vi "Multi-FuncGlobal.vi"(11 "Operation and Data In":T1) -> (1 "Time Out":dbl, 2 "Numeric Out":dbl, 3 "String Out":string)   [LabVIEW 2012]
doc: "This is a Multi-Functional Global Variable, meaning it can save a number, string, and also get the elapsed time since its time was last checked."
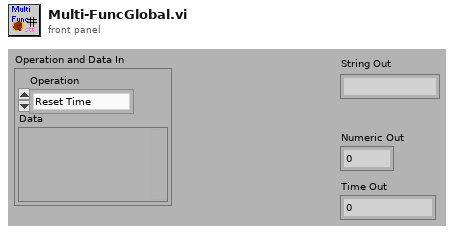
[diagram p1: front panel]
types:
  T1 = cluster{"Operation":enum16{"Reset Time", "Set String", "Set Number", "Get Elapsed Time", "Get String", "Get Number"}, "Data":variant}
  T2 = enum16{"Reset Time", "Set String", "Set Number", "Get Elapsed Time", "Get String", "Get Number"}
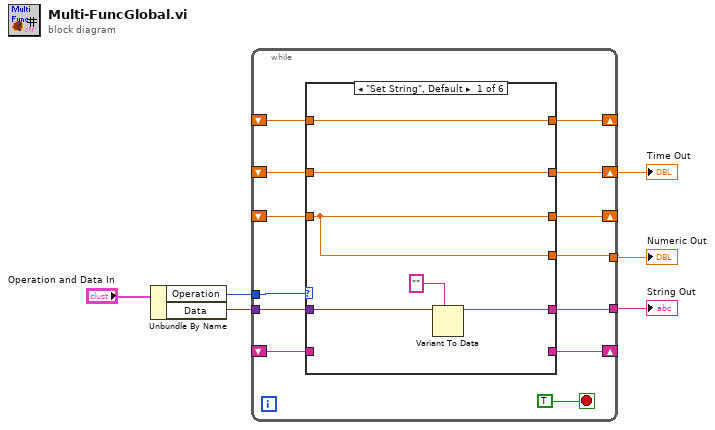
[diagram p0: block diagram]
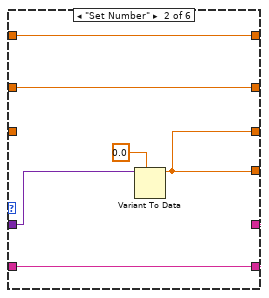
[diagram p2: hidden frame]
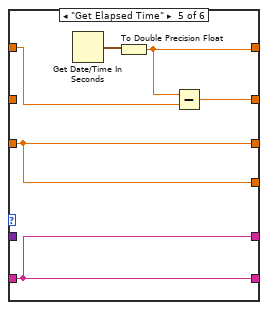
[diagram p5: hidden frame]
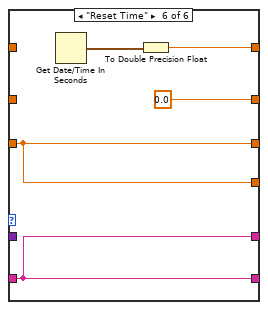
[diagram p6: hidden frame]
diagram:
  n1 = Unbundle By Name("Operation and Data In") -> ("Operation"=w5:T2, "Data"=w4:variant)
  n2 = while {
    tunnel: w5 -> [w19]
    tunnel: w4 -> [w18]
    tunnel: [w17] -> w3
    shift-right: [w15] -> _
    shift-left: _ -> [w14]
    tunnel: [w13] -> w2
    shift-right: [w12] -> _
    shift-left: _ -> [w11]
    shift-right: [w9] -> _
    shift-left: _ -> [w8]
    shift-right: [w10] -> w1
    shift-left: _ -> [w7]
    stop <- TRUE stop-if-true
    n3 = case shown="\"Set String\", Default" w19 {
      tunnel: w18 -> [w24 w31 _ _ _ _]
      tunnel: [w25 w29 w35 w39 w45 w50] -> w17
      tunnel: [w25 w29 w35 w39 w45 w50] -> w15
      tunnel: w14 -> [w25 _ w35 w39 w45 w50]
      tunnel: [w22 w28 w34 w38 w44 w49] -> w13
      tunnel: [w22 w28 w34 w38 w44 w49] -> w12
      tunnel: w11 -> [_ w28 w34 w38 w44 w49]
      tunnel: [w20 w26 w32 w36 w41 0.0 ("Time Out")] -> w10
      tunnel: [w21 w27 w33 w37 w40 w46] -> w9
      tunnel: w8 -> [w21 w27 w33 w37 w42 _]
      tunnel: w7 -> [w20 w26 w32 w36 _ _]
      frame "Set String", Default {
        n4 = Variant To Data(type="", Variant=w24) -> (data=w22:string)  [unwired: 1 in, 1 out]
      }
      frame "Set Number" {
        n5 = Variant To Data(type=0.0 ("Numeric Out"), Variant=w31) -> (data=w29:dbl)  [unwired: 1 in, 1 out]
      }
      frame "Get String" {
      }
      frame "Get Number" {
      }
      frame "Get Elapsed Time" {
        n6 = Get Date/Time In Seconds() -> (seconds since 1Jan1904=w43:timestamp)
        n7 = To Double Precision Float(number=w43) -> (double precision float=w40:dbl)
        n8 = Subtract(x=w40, y=w42) -> (x-y=w41:dbl)
      }
      frame "Reset Time" {
        n9 = Get Date/Time In Seconds() -> (seconds since 1Jan1904=w47:timestamp)
        n10 = To Double Precision Float(number=w47) -> (double precision float=w46:dbl)
      }
    }
  }
  "String Out" <- w2
  "Numeric Out" <- w3
  "Time Out" <- w1
